vi "asyncAcq_occRef_timeStamp_call_OSA200.vi"(0 "spectrIdx":u16, 3 "FTSLV.dll path":path, 5 "error in (no error)":errorcluster, 6 "timeStamp interferogram":u32, 8 "timeStamp spectrum":u32) -> (10 "timeStamp spectrum latest":u32, 12 "timeStamp interferogram latest":u32, 13 "error":i32, 16 "new spectrum":bool, 18 "new interferogram":bool, 19 "error out":errorcluster)   [LabVIEW 2010, in "OSA200.lvclass"]
doc: "SubVI to a <B>Thorlabs_OSA_64</B> object.\n\n[GOOP 1.0]"
uses:
  OSA200.lvclass
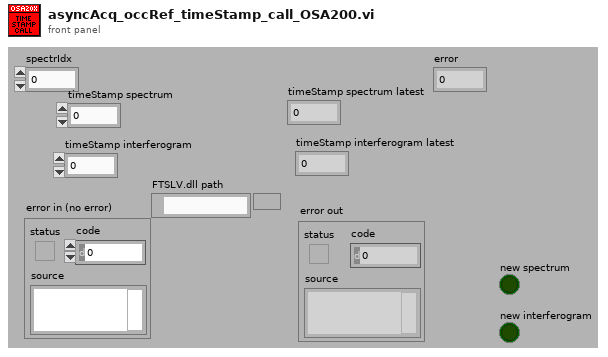
[diagram p1: front panel]
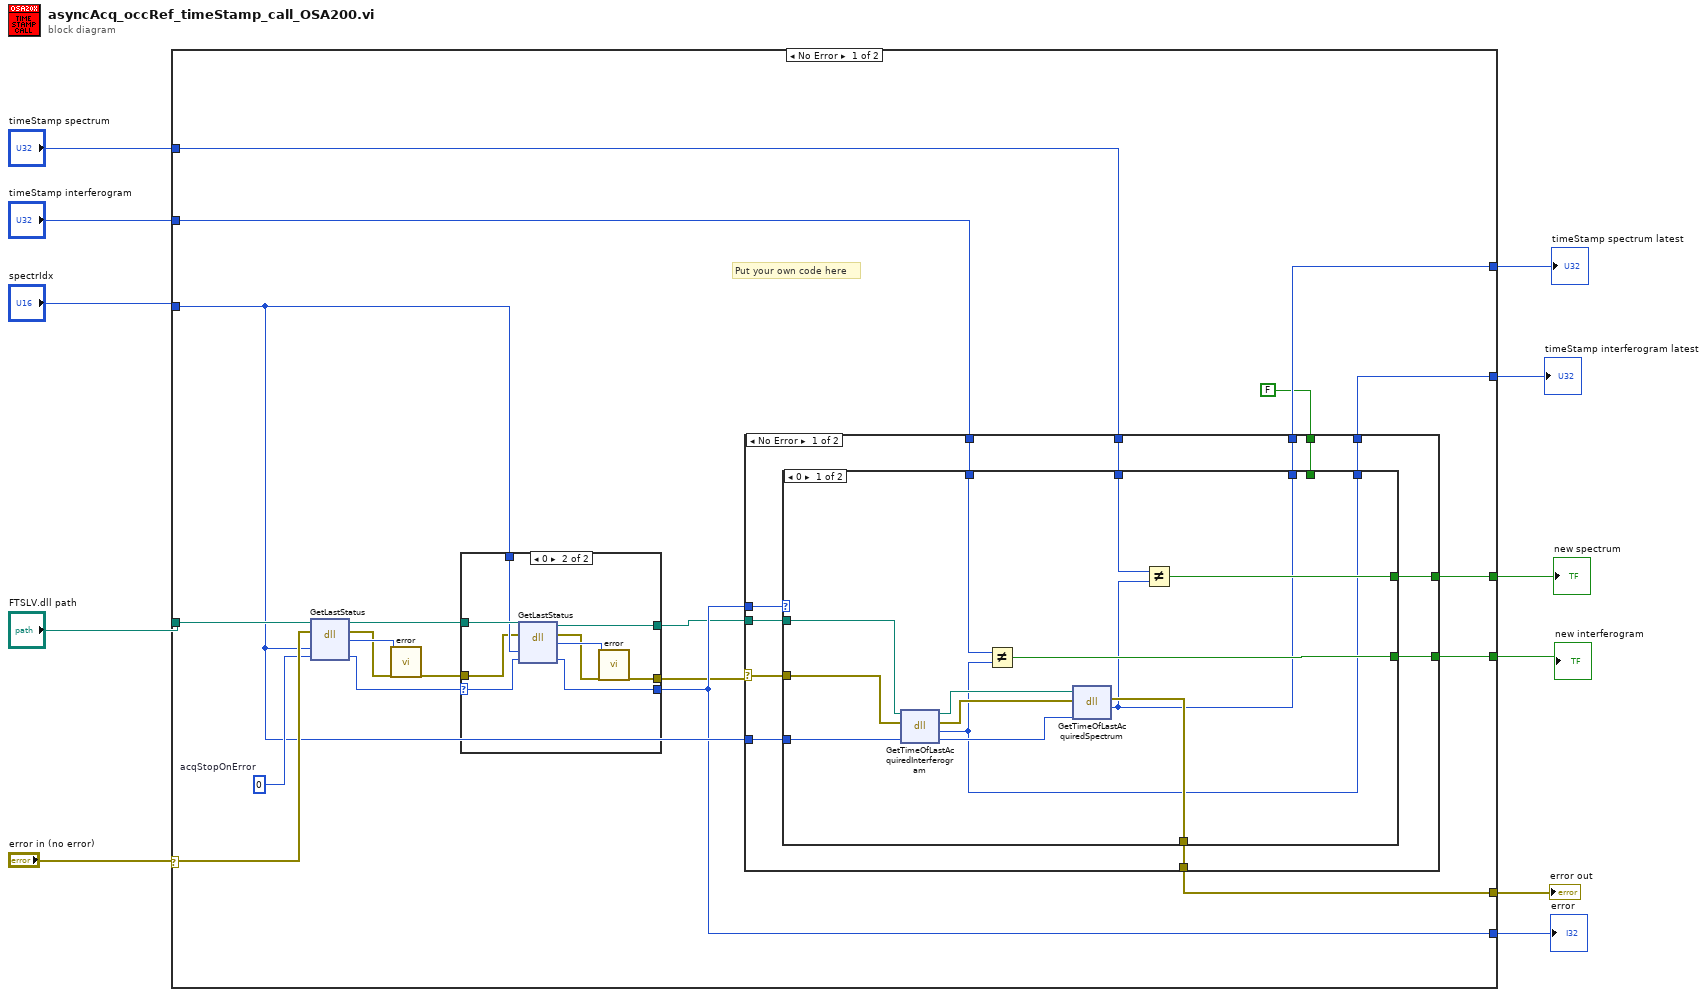
[diagram p0: block diagram]
diagram:
  n1 = case shown="No Error" "error in (no error)" {
    selector: "error in (no error)" -> [w25 w81]
    tunnel: [w22 w81] -> w11
    tunnel: "spectrIdx" -> [w15 _]
    tunnel: "timeStamp spectrum" -> [w31 w79]
    tunnel: "timeStamp interferogram" -> [w30 w80]
    tunnel: [w29 w79] -> w6
    tunnel: [w28 w80] -> w5
    tunnel: [w27 w78] -> w4
    tunnel: [w26 w78] -> w3
    tunnel: [w14 u8 0 ("acqStopOnError")] -> w2
    tunnel: "FTSLV.dll path" -> [w23 _]
    frame No Error {
      w21 = 0  # acqStopOnError
      # "Put your own code here"
      n2 = dll-call lib="?" fn="GetLastStatus" ("Thorlabs_FTS_asynchAcq.dll:Thorlabs_FTS_asynchAcq_handle")(path in=w23, error in=w25, "spectrIdx"=w15, "acqStopOnError"=w21) -> (path out=w16:path, error out=w19:errorcluster, "return type"=w20:u32, "acqStopOnError"=w18:i32)  [unwired: 2 in]
      n3 = call "error.vi"("result code"=w20, "error in (no error)"=w19) -> ("error out"=w17:errorcluster)  [unwired: 15 in, 2 out]
      n4 = case shown="0" w18 {
        selector: w18 -> [w34 w37]
        tunnel: w17 -> [w32 w38]
        tunnel: w16 -> [w33 w41]
        tunnel: [w33 w40] -> w13
        tunnel: w15 -> [_ w39]
        tunnel: [w34 w36] -> w14
        tunnel: [w32 w35] -> w12
        frame Default {
        }
        frame 0 {
          n5 = dll-call lib="?" fn="GetLastStatus" ("Thorlabs_FTS_asynchAcq.dll:Thorlabs_FTS_asynchAcq_handle")(path in=w41, error in=w38, "spectrIdx"=w39, "acqStopOnError"=w37) -> (path out=w40:path, error out=w42:errorcluster, "return type"=w43:u32, "acqStopOnError"=w36:i32)  [unwired: 2 in]
          n6 = call "error.vi"("result code"=w43, "error in (no error)"=w42) -> ("error out"=w35:errorcluster)  [unwired: 15 in, 2 out]
        }
      }
      n7 = case shown="No Error" w12 {
        selector: w12 -> [w45 w73]
        tunnel: w15 -> [w55 _]
        tunnel: w31 -> [w54 w76]
        tunnel: w30 -> [w52 w75]
        tunnel: [w53 w74] -> w27
        tunnel: [w51 w74] -> w26
        tunnel: [w50 w76] -> w29
        tunnel: [w49 w75] -> w28
        tunnel: w14 -> [w48 _]
        tunnel: FALSE -> [w47 w74]
        tunnel: w13 -> [w46 _]
        tunnel: [w44 w73] -> w22
        frame No Error {
          n8 = case shown="0" w48 {
            tunnel: w55 -> [w68 _]
            tunnel: w54 -> [w62 w72]
            tunnel: [w60 w70] -> w53
            tunnel: w52 -> [w56 w71]
            tunnel: [w59 w70] -> w51
            tunnel: [w58 w72] -> w50
            tunnel: [w57 w71] -> w49
            tunnel: w47 -> [_ w70]
            tunnel: w46 -> [w66 _]
            tunnel: w45 -> [w64 w69]
            tunnel: [w61 w69] -> w44
            frame 0 {
              n9 = dll-call lib="?" fn="GetTimeOfLastAcquiredInterferogram" ("Thorlabs_FTS_asynchAcq.dll:Thorlabs_FTS_asynchAcq_handle")(path in=w66, error in=w64, "spectrIdx"=w68) -> (path out=w65:path, error out=w63:errorcluster, "return type"=w57:u32, "spectrIdx"=w67:u16)  [unwired: 1 in]
              n10 = Not Equal?(x=w56, y=w57) -> (x != y?=w59:bool)
              n11 = dll-call lib="?" fn="GetTimeOfLastAcquiredSpectrum" ("Thorlabs_FTS_asynchAcq.dll:Thorlabs_FTS_asynchAcq_handle")(path in=w65, error in=w63, "spectrIdx"=w67) -> (error out=w61:errorcluster, "return type"=w58:u32)  [unwired: 2 in, 1 out]
              n12 = Not Equal?(x=w62, y=w58) -> (x != y?=w60:bool)
            }
            frame Default {
            }
          }
        }
        frame Error {
        }
      }
    }
    frame Error {
      w78 = FALSE
      # "Error"
    }
  }
  "error out" <- w11
  "timeStamp interferogram latest" <- w5
  "timeStamp spectrum latest" <- w6
  "new spectrum" <- w4
  "new interferogram" <- w3
  "error" <- w2
